vi "Set_Thermistor_Offset.vi"() -> ()   [LabVIEW 2016]
uses:
  Sub VIs/ADAM Controls/Channel_names.ctl
  Sub VIs/ADAM Controls/Module_type_ADAM.ctl
  Sub VIs/ADAM Controls/Calib_type_ADAM.ctl
  <vilib>/Analysis/baseanly.llb/Mean (DBL).vi
  <vilib>/Analysis/NI_AALBase.lvlib
panel:
  in  "Apply Offset":bool
  in  "Stop Looping":bool
  out "Offsets needed":dbl[](array[numeric])
  out "Waveform Graph":dbl[][](graph)
  in  "History Length (mins)":dbl=2.0
  out "Selected Channel Names":string[](array[string])
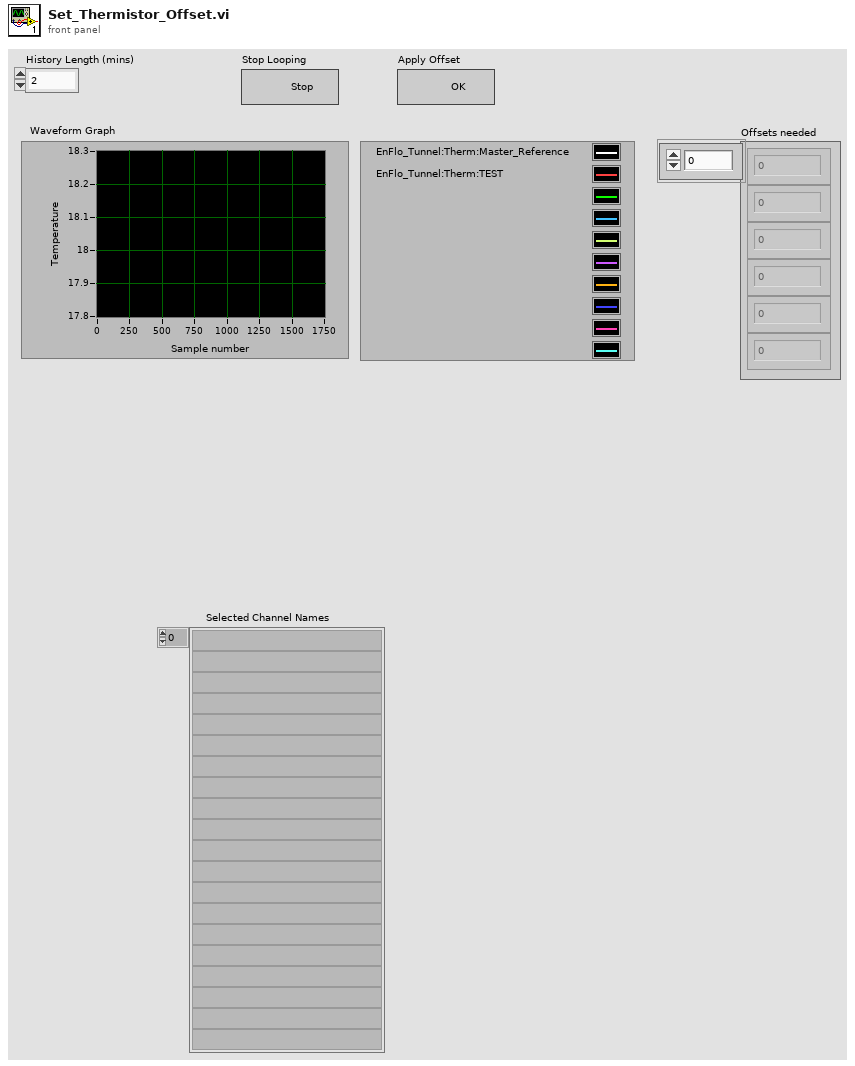
[diagram p1: front panel]
types:
  T1 = enum16{"Zero or one", "One", "Zero or more", "One or more"}
  T2 = typedef "Channel_names.ctl" = enum16{"Active Only", "Active + Off", "All Channels"}
  T3 = typedef "Module_type_ADAM.ctl" = string
  T4 = typedef "Calib_type_ADAM.ctl" = enum16{"Raw", "Bx + A", "Cx^2 + Bx + A", "Dx^3 + Cx^2 + Bx + A", "In Band", "Hi-Tec Q", "Hi-Tec M_dot", "Text"}
  T5 = typedef "Ch_description_ADAM.ctl" = cluster{"Ch Name":string, "Type":T3, "Function":T6, "Ch State":T7, "Calibration type":T4, "A":dbl, "B":dbl, "C":dbl, "D":dbl, "Comments":string, "Address":T8, "String":string, "Duty":u16}
  T6 = typedef "Function_ADAM.ctl" = enum16{"Analogue Input", "Digital Input", "Event counter", "Event rate", "Analogue Output", "Digital Output", "Relay Output"}
  T7 = typedef "Channel_State.ctl" = enum16{"On", "Off", "Always On", "Always Off"}
  T8 = typedef "Address.ctl" = cluster{"Main":i32, "Ch.":i32, "Sub":i32, "Port Name":string}
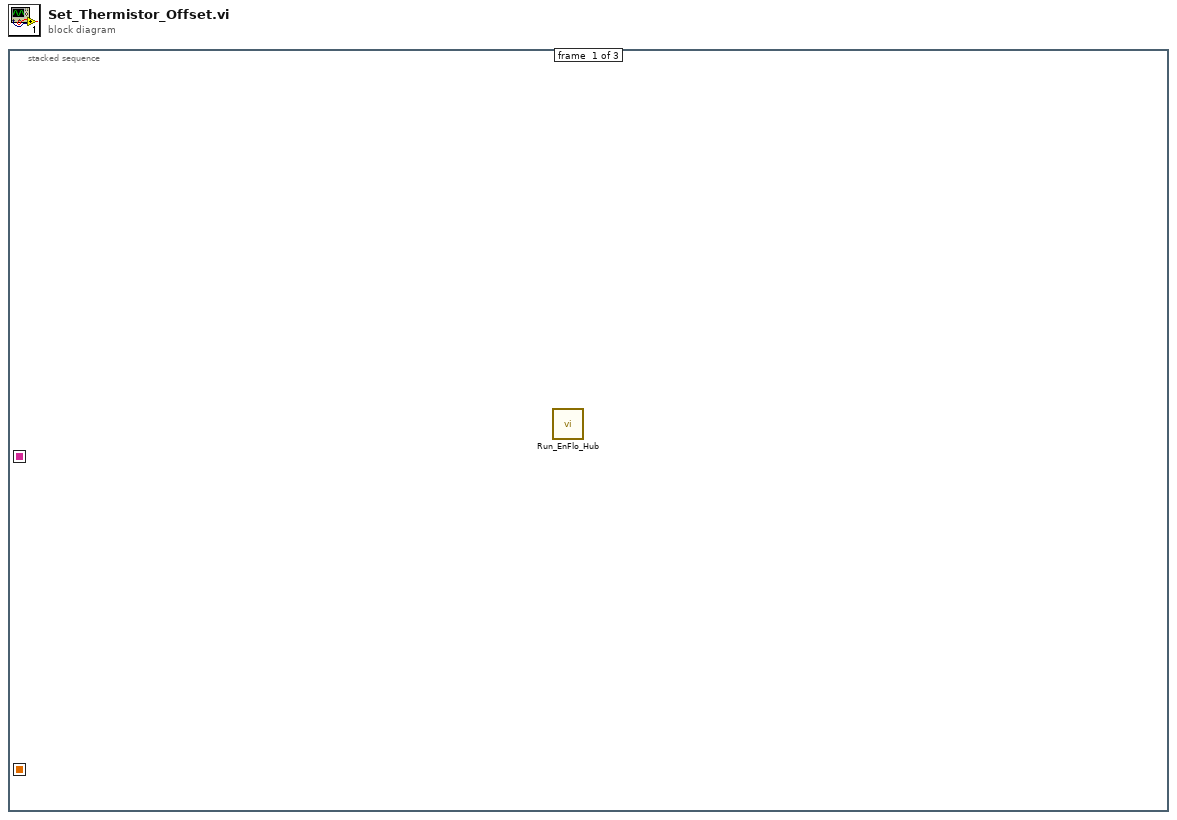
[diagram p0: block diagram]
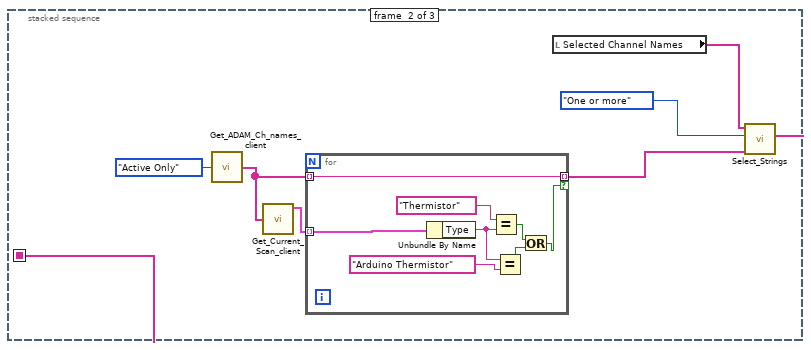
[diagram p2: hidden frame]
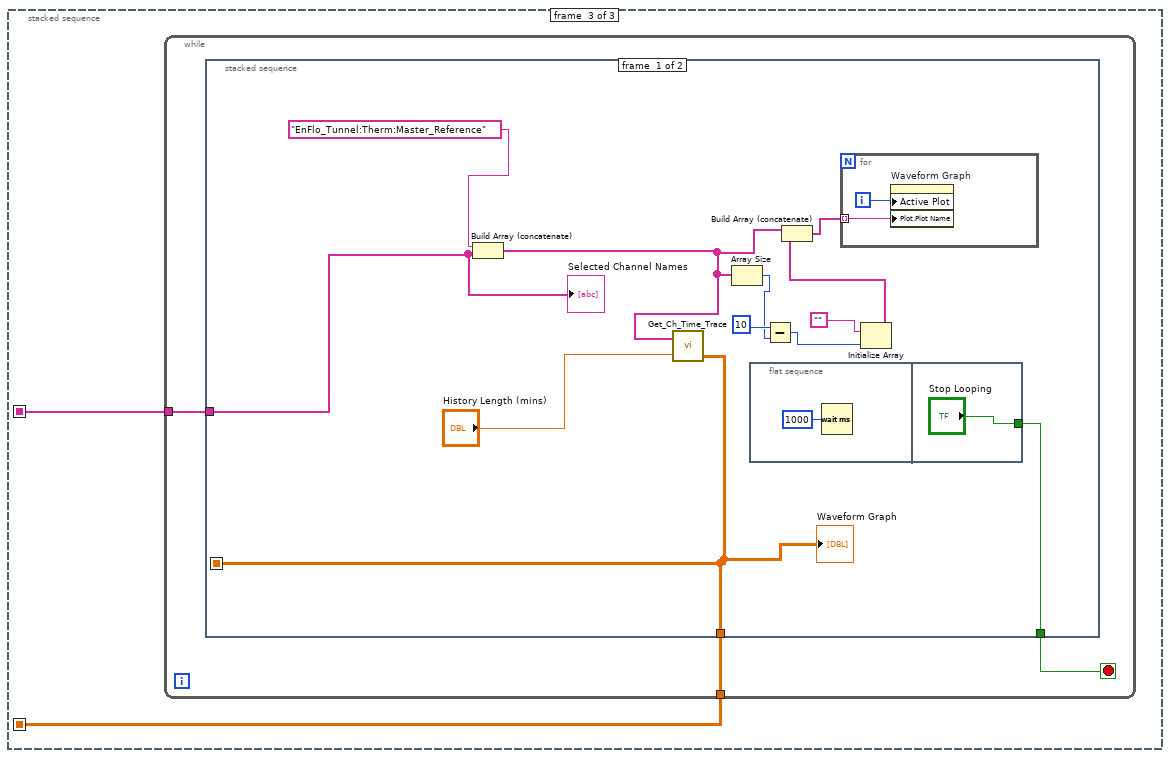
[diagram p3: hidden frame]
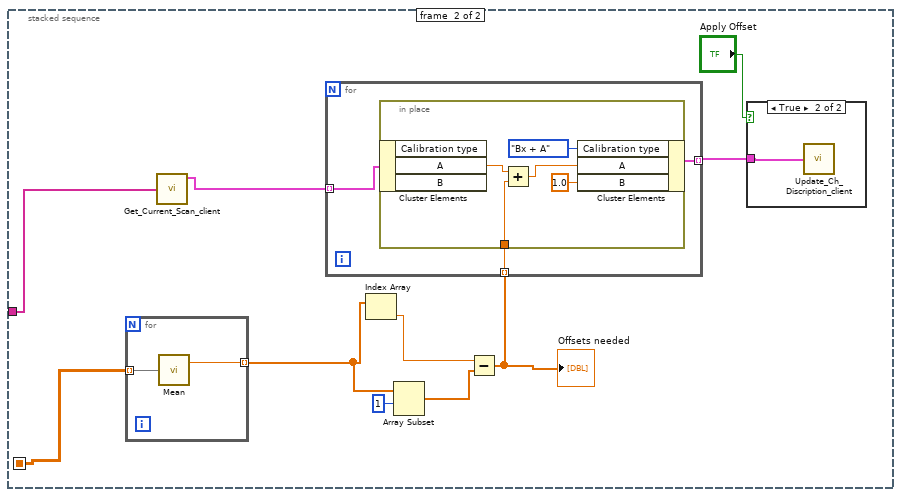
[diagram p4: hidden frame]
diagram:
  n1 = stacked-sequence {
    seq-local: [_ _ w17] -> [_ _ _]
    seq-local: [_ w1 _] -> [_ _ w16]
    frame #0 {
      n2 = call "Run_EnFlo_Hub.vi"() -> ()  [unwired: 7 in, 1 out]
    }
    frame #1 {
      n3 = call "Get_ADAM_Ch_names_client.vi"("Channel names set"=Channel_names."Active Only") -> ("Ch names"=w2:string[])
      n4 = call "Get_Current_Scan_client.vi"("ADAM Ch Names"=w2) -> ("Ch Description Array"=w4:T5[])  [unwired: 1 in, 2 out]
      n5 = for {
        tunnel: w4 -> [w15] mode=indexing
        tunnel: [w9] -> w3 mode=indexing if=w8
        tunnel: w2 -> [w9] mode=indexing
        n6 = Unbundle By Name(w15) -> ("Type"=w13:T3)
        n7 = Equal?(x=T3 "Thermistor" ("Type"), y=w13) -> (x = y?=w11:bool)
        n8 = Equal?(x=w13, y=T3 "Arduino Thermistor" ("Type")) -> (x = y?=w10:bool)
        n9 = Or(x=w11, y=w10) -> (x .or. y?=w8:bool)
      }
      n10 = local read "Selected Channel Names"() -> (w5:string[])
      n11 = call "Select_Strings.vi"("Available Ch names"=w3, "Selector mode"=T1."One or more", "Desired Ch names (in)"=w5) -> ("Selected Channel Names"=w1:string[])  [unwired: 3 in, 2 out]
    }
    frame #2 {
      n12 = while {
        tunnel: [w20] -> w17
        tunnel: w16 -> [w19]
        stop <- w18 stop-if-true
        n13 = stacked-sequence {
          seq-local: [w28 _] -> [_ w41]
          tunnel: [w28 _] -> w20
          tunnel: w19 -> [w30 w37]
          tunnel: [w29 _] -> w18
          frame #0 {
            n14 = Build Array (concatenate)("EnFlo_Tunnel:Therm:Master_Reference", w30) -> (w24:string[])
            n15 = call "Get_Ch_Time_Trace.vi"("Desired Ch Names"=w24, "History Length (mins)"="History Length (mins)") -> ("Output array"=w28:dbl[][])  [unwired: 2 out]
            "Waveform Graph" <- w28
            n16 = Array Size(array=w24) -> (size(s)=w22:i32)
            n17 = flat-sequence {
              tunnel: ["Stop Looping"] -> w29
              frame #0 {
                n18 = Wait (ms)(milliseconds to wait=u32 1000) -> ()  [unwired: 1 out]
              }
              frame #1 {
              }
            }
            n19 = Subtract(x=10 ("dimension size"), y=w22) -> (x-y=w21:i32)
            n20 = Initialize Array("", w21) -> (w25:string[])
            n21 = Build Array (concatenate)(w24, w25) -> (w26:string[])
            n22 = for {
              tunnel: w26 -> [w35] mode=indexing
              i -> [w36]
              n23 = property on="Waveform Graph" class="WFGraph (strict)"("Active Plot"=w36, "Plot.Plot Name"=w35) -> ()  [unwired: 2 in, 2 out]
            }
            "Selected Channel Names" <- w30
          }
          frame #1 {
            n24 = for {
              tunnel: w41 -> [w49] mode=indexing
              tunnel: [w48] -> w40 mode=indexing
              n25 = call-poly <vilib>:"Mean.vi"("X"=w49) -> ("mean"=w48:dbl)  [unwired: 1 out]
            }
            n26 = call "Get_Current_Scan_client.vi"("ADAM Ch Names"=w37) -> ("Ch Description Array"=w43:T5[])  [unwired: 1 in, 2 out]
            n27 = Index Array(array=w40) -> (element=w45:dbl)  [unwired: 1 in]
            n28 = Array Subset(array=w40, index=1) -> (w44:dbl[])  [unwired: 1 in]
            n29 = Subtract(x=w45, y=w44) -> (x-y=w42:dbl[])
            "Offsets needed" <- w42
            n30 = for {
              tunnel: w43 -> [w52] mode=indexing
              tunnel: w42 -> [w51] mode=indexing
              tunnel: [w50] -> w39 mode=indexing
              n31 = in-place {
                in-place-border: w51 -> [w56]
                n32 = in-place-cluster #1(w52) -> ("A"=w57:dbl)  [unwired: 2 out]
                n33 = Add(x=w57, y=w56) -> (x+y=w55:dbl)
                n34 = in-place-cluster #1("Calibration type"=Calib_type_ADAM."Bx + A", "A"=w55, "B"=1.0) -> (w50:T5)
              }
            }
            n35 = case shown="True" "Apply Offset" {
              tunnel: w39 -> [_ w47]
              frame False {
              }
              frame True {
                n36 = call "Update_Ch_Discription_client.vi"("Channels to update In"=w47) -> ()  [unwired: 1 in]
              }
            }
          }
        }
      }
    }
  }
